vi "Set Index.vi"(8 "error in":errorcluster, 10 "Index":u16 format="%.0x", 11 "Object Entry in":refnum<class "Object Entry.lvclass">) -> (0 "error out":errorcluster, 3 "Object Entry out":refnum<class "Object Entry.lvclass">)   [LabVIEW 2019, in "Electronic Datasheet.lvlib" / "Object Entry.lvclass"]
uses:
  Object Entry.lvclass
  Object Entry.lvclass/Object Entry.ctl
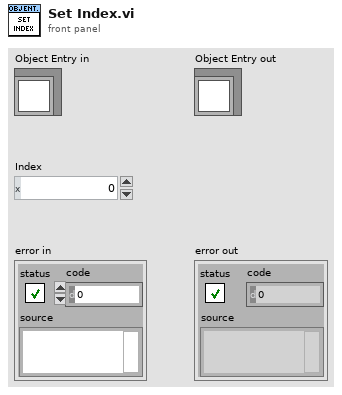
[diagram p1: front panel]
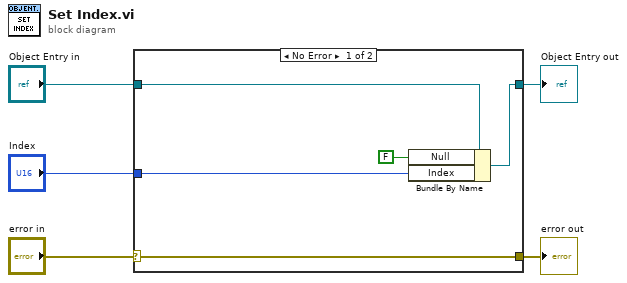
[diagram p0: block diagram]
diagram:
  n1 = case shown="No Error" "error in" {
    selector: "error in" -> [w10 w11]
    tunnel: [w10 w11] -> w4
    tunnel: [w8 w12] -> w2
    tunnel: "Object Entry in" -> [w9 w12]
    tunnel: "Index" -> [w7 _]
    frame No Error {
      n2 = Bundle By Name(cluster=w9, "Null"=FALSE ("Index.Null"), "Index"=w7) -> (w8:refnum<class "Object Entry.lvclass">)
    }
    frame Error {
    }
  }
  "error out" <- w4
  "Object Entry out" <- w2
